vi "Rinocloud_local_mirror.vi"(6 "Store metadata":bool, 7 "ancestor array":T1(array[cluster]), 8 "error in":errorcluster, 9 "JSON payload":string, 10 "file name":string, 11 "file path":path) -> (0 "error out":errorcluster)   [LabVIEW 2011, in "Rinocloud Library.lvlib"]
uses:
  Rinocloud Library.lvlib
  Rinocloud_global_variable.vi
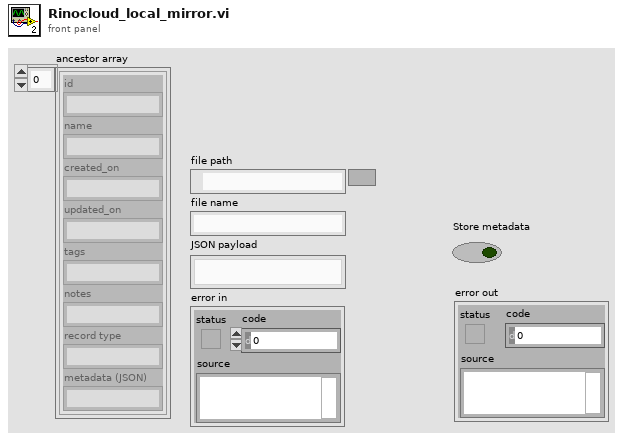
[diagram p1: front panel]
types:
  T1 = cluster{"id":string, "name":string, "created_on":string, "updated_on":string, "tags":string, "notes":string, "record type":string, "metadata (JSON)":string}[]
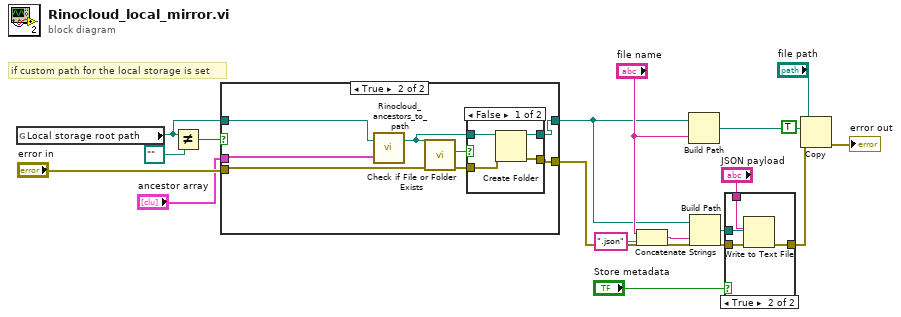
[diagram p0: block diagram]
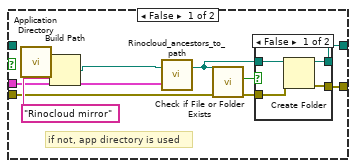
[diagram p3: hidden frame]
diagram:
  # "if custom path for the local storage is set"
  n1 = global read "Rinocloud_global_variable.vi" "Local storage root path"() -> (w11:path)
  n2 = Not Equal?(x=w11, y=path "") -> (x != y?=w12:bool)
  n3 = case shown="True" w12 {
    tunnel: w11 -> [_ w38]
    tunnel: [w24 w37] -> w3
    tunnel: [w23 w36] -> w10
    tunnel: "error in" -> [w22 w39]
    tunnel: "ancestor array" -> [w19 w35]
    frame False {
      # "if not, app directory is used"
      n4 = call <vilib>:"Application Directory.vi"() -> ("Application Directory"=w25:path)
      n5 = Build Path(base path=w25, name or relative path="Rinocloud mirror") -> (appended path=w21:path)
      n6 = call "Rinocloud_ancestors_to_path.vi"("ancestor array"=w19, "Path"=w21) -> ("full path"=w20:path)  [unwired: 1 in]
      n7 = call <vilib>:"Check if File or Folder Exists.vi"("error in (no error)"=w22, "path"=w20) -> ("error out"=w28:errorcluster, "file or folder exists?"=w27:bool)  [unwired: 7 in, 1 out]
      n8 = case shown="False" w27 {
        tunnel: [w29 w34] -> w24
        tunnel: w20 -> [w32 w34]
        tunnel: w28 -> [w31 w33]
        tunnel: [w30 w33] -> w23
        frame False {
          n9 = Create Folder(path (use dialog)=w32, error in=w31) -> (created path=w29:path, error out=w30:errorcluster)  [unwired: 1 in, 1 out]
        }
        frame True {
        }
      }
    }
    frame True {
      n10 = call "Rinocloud_ancestors_to_path.vi"("ancestor array"=w35, "Path"=w38) -> ("full path"=w40:path)  [unwired: 1 in]
      n11 = call <vilib>:"Check if File or Folder Exists.vi"("error in (no error)"=w39, "path"=w40) -> ("error out"=w42:errorcluster, "file or folder exists?"=w41:bool)  [unwired: 7 in, 1 out]
      n12 = case shown="False" w41 {
        tunnel: [w43 w48] -> w37
        tunnel: w40 -> [w46 w48]
        tunnel: w42 -> [w45 w47]
        tunnel: [w44 w47] -> w36
        frame False {
          n13 = Create Folder(path (use dialog)=w46, error in=w45) -> (created path=w43:path, error out=w44:errorcluster)  [unwired: 1 in, 1 out]
        }
        frame True {
        }
      }
    }
  }
  n14 = Concatenate Strings("file name", ".json" ("string")) -> (w15:string)
  n15 = Build Path(base path=w3, name or relative path="file name") -> (appended path=w17:path)
  n16 = Build Path(base path=w3, name or relative path=w15) -> (appended path=w14:path)
  n17 = case shown="True" "Store metadata" {
    tunnel: w14 -> [_ w53]
    tunnel: [w49 w52] -> w13
    tunnel: w10 -> [w49 w51]
    tunnel: "JSON payload" -> [_ w50]
    frame False {
    }
    frame True {
      n18 = Write to Text File(file (use dialog)=w53, text=w50, error in=w51) -> (error out=w52:errorcluster)  [unwired: 1 in, 2 out]
    }
  }
  n19 = Copy(8:w13, 9:TRUE ("overwrite (F)"), 10:w17, 11:"file path") -> (0:→"error out":errorcluster)  [unwired: 1 in, 2 out]
